vi "Config Paths.vi"(8 "error in (no error)":errorcluster) -> (0 "error out":errorcluster, 1 "Process Config":path, 2 "Preset Config":path, 3 "Global Config":path)   [LabVIEW 2017]
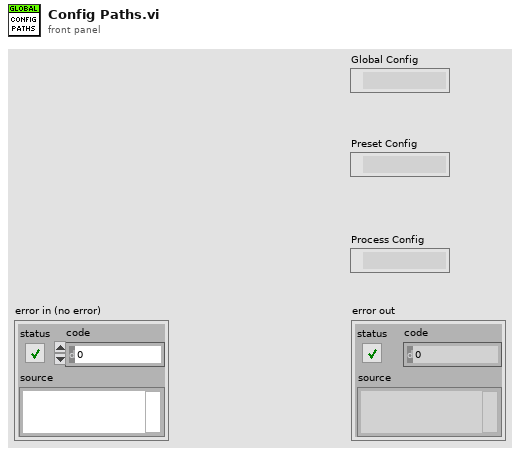
[diagram p1: front panel]
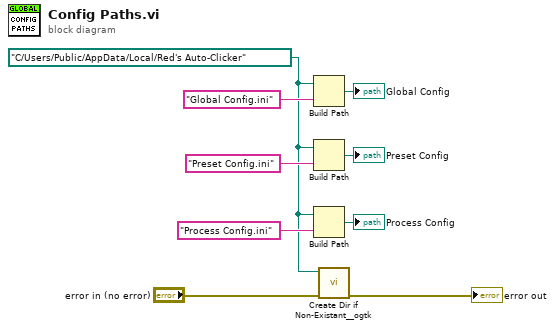
[diagram p0: block diagram]
diagram:
  w1 = path "C:/Users/Public/AppData/Local/Red's Auto-Clicker"
  n1 = Build Path(base path=w1, name or relative path="Global Config.ini") -> (appended path=→"Global Config":path)
  n2 = Build Path(base path=w1, name or relative path="Preset Config.ini") -> (appended path=→"Preset Config":path)
  n3 = Build Path(base path=w1, name or relative path="Process Config.ini") -> (appended path=→"Process Config":path)
  n4 = call <userlib>:"Create Dir if Non-Existant__ogtk.vi"("error in (no error)"="error in (no error)", "Directory Path"=w1) -> ("error out"=→"error out":errorcluster)  [unwired: 7 in, 2 out]
